vi "COD_所有参数读取.vi"(8 "error in (no error)":errorcluster caption="错误输入（无错误）", 11 "MB session in":refnum<class "MB_Master.lvclass">) -> (0 "error out":errorcluster caption="错误输出", 2 "输出值":T1 {"电极型号标志" items=["NULL"=0, "pH"=1, "Cond"=2, "DO"=3, "Turb"=4, "COD"=8]; "电极状态标志" items=["OK"=0, "温湿度报警"=7, "马达故障"=31]}, 3 "MB session out":refnum<class "MB_Master.lvclass">)   [LabVIEW 2016, in "斯坦道多参数.lvlib"]
uses:
  <vilib>/Plasmionique/MB Master/MB_Master/MB_Master.lvclass
  <vilib>/Plasmionique/MB Master/MB Master.lvlib
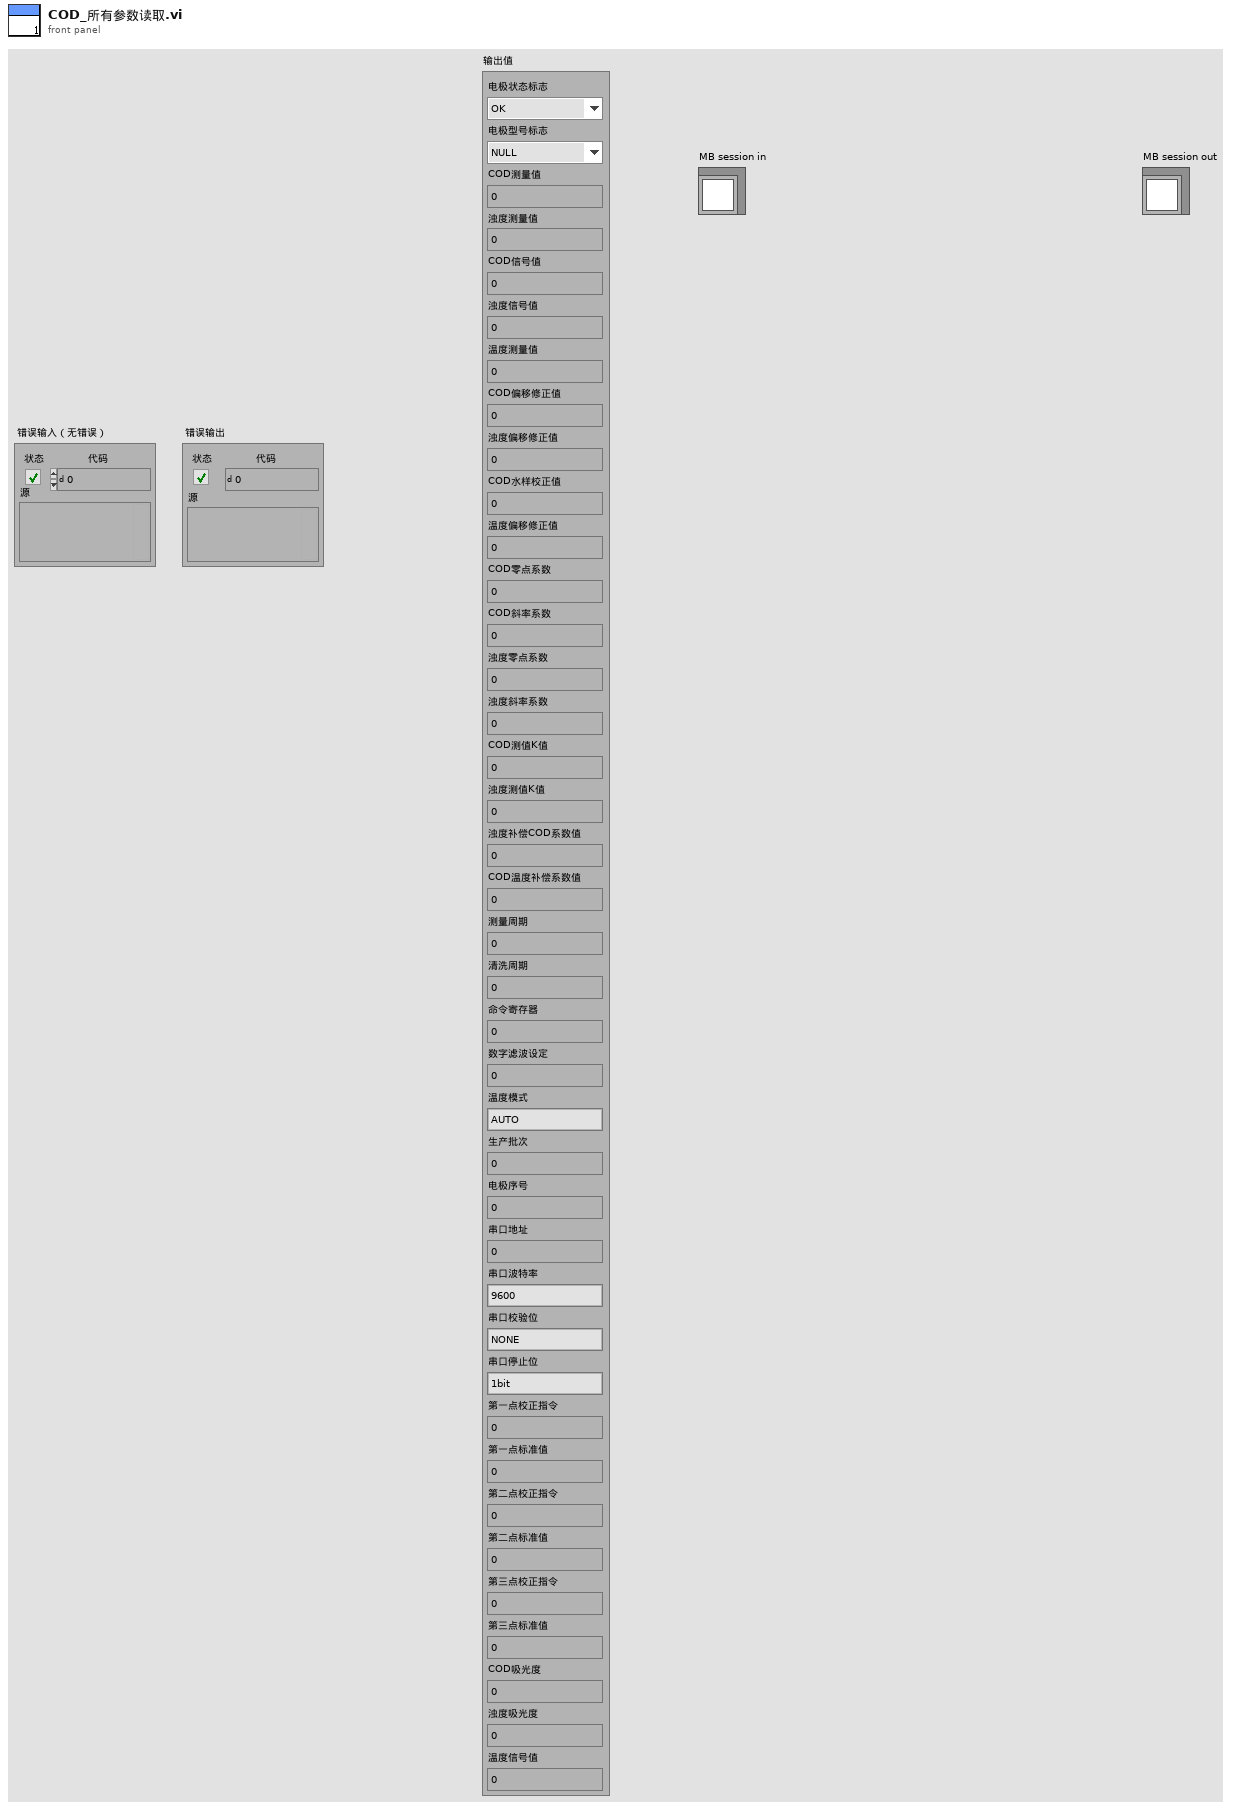
[diagram p1: front panel]
types:
  T1 = cluster{"电极状态标志":u16, "电极型号标志":u16, "COD测量值":sgl, "浊度测量值":sgl, "COD信号值":sgl, "浊度信号值":sgl, "温度测量值":sgl, "COD偏移修正值":sgl, "浊度偏移修正值":sgl, "COD水样校正值":sgl, "温度偏移修正值":sgl, "COD零点系数":sgl, "COD斜率系数":sgl, "浊度零点系数":sgl, "浊度斜率系数":sgl, "COD测值K值":sgl, "浊度测值K值":sgl, "浊度补偿COD系数值":sgl, "COD温度补偿系数值 ":sgl, "测量周期":u16, "清洗周期":u16, "命令寄存器":u16, "数字滤波设定":u16, "温度模式":enum16{"AUTO", "OFF"}, "生产批次":u16, "电极序号":u16, "串口地址":u16, "串口波特率":enum16{"9600", "19200", "115200"}, "串口校验位":enum16{"NONE", "ODD", "EVEN"}, "串口停止位":enum16{"1bit", "2bit"}, "第一点校正指令":u16, "第一点标准值":sgl, "第二点校正指令":u16, "第二点标准值":sgl, "第三点校正指令":u16, "第三点标准值":sgl, "COD吸光度":sgl, "浊度吸光度":sgl, "温度信号值":sgl}
  T2 = cluster{u16, u16, "数值":sgl, "数值":sgl, "数值":sgl, "数值":sgl, "数值":sgl, "数值":sgl, "数值":sgl, "数值":sgl, "数值":sgl, "数值":sgl, "数值":sgl, "数值":sgl, "数值":sgl, "数值":sgl, "数值":sgl, "数值":sgl, "数值":sgl, u16, u16, u16, u16, u16, u16, u16, u16, u16, u16, u16, u16, "数值":sgl, u16, "数值":sgl, u16, "数值":sgl, "数值":sgl, "数值":sgl, "数值":sgl}
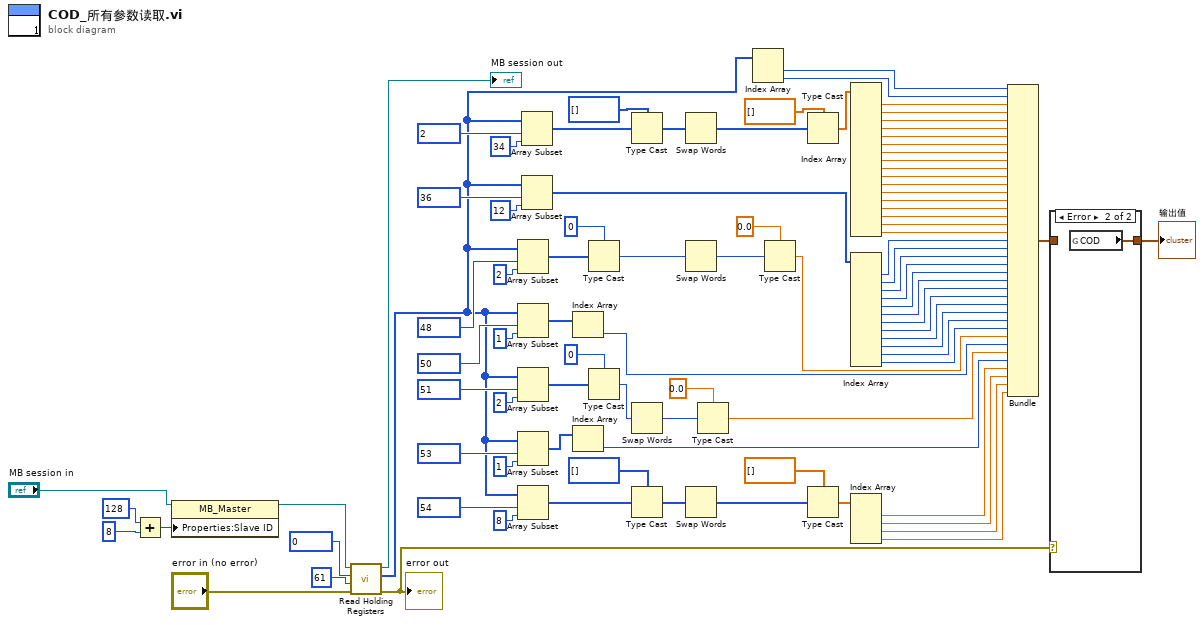
[diagram p0: block diagram]
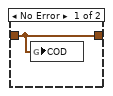
[diagram p2: hidden frame]
diagram:
  n1 = Add(x=u16 128, y=u16 8) -> (x+y=w91:u16)
  n2 = property class="MB_Master"(reference="MB session in", "Properties:Slave ID"=w91) -> (reference out=w49:refnum<class "MB_Master.lvclass">)  [unwired: 1 in, 1 out]
  n3 = call <vilib>:"Read Holding Registers.vi"("error in (no error)"="error in (no error)", "quantity"=u16 61, "starting address"=u16 0, "MB session in"=w49) -> ("error out"=w48:errorcluster, "Registers"=w15:u16[], "MB session out"=→"MB session out":refnum<class "MB_Master.lvclass">)  [unwired: 5 in]
  "error out" <- w48
  n4 = Array Subset(array=w15, index=u16 48 ("starting address"), length=2 ("长度")) -> (w56:u16[])
  n5 = Array Subset(array=w15, index=u16 50 ("starting address"), length=1 ("长度")) -> (w14:u16[])
  n6 = Array Subset(array=w15, index=u16 51 ("starting address"), length=2 ("长度")) -> (w51:u16[])
  n7 = Array Subset(array=w15, index=u16 53 ("starting address"), length=1 ("长度")) -> (w12:u16[])
  n8 = Array Subset(array=w15, index=u16 54 ("starting address"), length=8 ("长度")) -> (w47:u16[])
  n9 = Array Subset(array=w15, index=u16 2 ("starting address"), length=34 ("长度")) -> (w80:u16[])
  n10 = Array Subset(array=w15, index=u16 36 ("starting address"), length=12 ("长度")) -> (w73:u16[])
  n11 = Index Array(array=w14) -> (element=w4:u16)  [unwired: 1 in]
  n12 = Index Array(array=w12) -> (element=w3:u16)  [unwired: 1 in]
  n13 = Type Cast(type=u32 0 ("数值"), x=w56) -> (*(type *) &x=w59:u32)
  n14 = Type Cast(type=u32 0 ("数值"), x=w51) -> (*(type *) &x=w53:u32)
  n15 = Type Cast(type=u32[] [] ("数组 2"), x=w80) -> (*(type *) &x=w82:u32[])
  n16 = Swap Words(1:w53) -> (0:w52:u32)
  n17 = Type Cast(type=u32[] [] ("数组 2"), x=w47) -> (*(type *) &x=w45:u32[])
  n18 = Swap Words(1:w82) -> (0:w84:u32[])
  n19 = Swap Words(1:w59) -> (0:w60:u32)
  n20 = Swap Words(1:w45) -> (0:w46:u32[])
  n21 = Type Cast(type=sgl 0.0 ("数值"), x=w52) -> (*(type *) &x=w13:sgl)
  n22 = Index Array(array=w15) -> (element #1=w87:u16, element #2=w86:u16)  [unwired: 2 in]
  n23 = Type Cast(type=sgl 0.0 ("数值"), x=w60) -> (*(type *) &x=w20:sgl)
  n24 = Type Cast(type=sgl[] [] ("数组 2"), x=w84) -> (*(type *) &x=w79:sgl[])
  n25 = Type Cast(type=sgl[] [] ("数组 2"), x=w46) -> (*(type *) &x=w9:sgl[])
  n26 = Index Array(array=w79) -> (element #1=w40:sgl, element #2=w78:sgl, element #3=w77:sgl, element #4=w38:sgl, element #5=w37:sgl, element #6=w36:sgl, element #7=w35:sgl, element #8=w34:sgl, element #9=w33:sgl, element #10=w32:sgl, element #11=w31:sgl, element #12=w30:sgl, element #13=w29:sgl, element #14=w28:sgl, element #15=w27:sgl, element #16=w26:sgl, element #17=w25:sgl)  [unwired: 17 in]
  n27 = Index Array(array=w73) -> (element #1=w72:u16, element #2=w71:u16, element #3=w70:u16, element #4=w69:u16, element #5=w68:u16, element #6=w67:u16, element #7=w66:u16, element #8=w65:u16, element #9=w24:u16, element #10=w23:u16, element #11=w22:u16, element #12=w21:u16)  [unwired: 12 in]
  n28 = Index Array(array=w9) -> (element #1=w8:sgl, element #2=w7:sgl, element #3=w6:sgl, element #4=w5:sgl)  [unwired: 4 in]
  n29 = Bundle(w87, w86, "数值"=w40, "数值"=w78, "数值"=w77, "数值"=w38, "数值"=w37, "数值"=w36, "数值"=w35, "数值"=w34, "数值"=w33, "数值"=w32, "数值"=w31, "数值"=w30, "数值"=w29, "数值"=w28, "数值"=w27, "数值"=w26, "数值"=w25, w72, w71, w70, w69, w68, w67, w66, w65, w24, w23, w22, w21, "数值"=w20, w4, "数值"=w13, w3, "数值"=w8, "数值"=w7, "数值"=w6, "数值"=w5) -> (w2:T2)  [unwired: 1 in]
  n30 = case shown="Error" w48 {
    tunnel: w2 -> [w92 _]
    tunnel: [w92 w93] -> w1
    frame No Error {
      n31 = global write "国弘过程全局变量.vi" "COD"(w92) -> ()
    }
    frame Error {
      n32 = global read "国弘过程全局变量.vi" "COD"() -> (w93:T1)
    }
  }
  "输出值" <- w1
